vi "Generate Callchain.vi"() -> (3 "Callchain":string)   [LabVIEW 2020, in "hse-logger.lvlib" / "LogRecord.lvclass"]
doc: "Generates a easy to read callchain. Entries from the hse-logger.lvlib are ignored.\n\n____\nHAMPEL SOFTWARE ENGINEERING v2.0.6 (2021-04-15 11:38)"
uses:
  LogRecord.lvclass
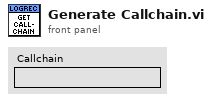
[diagram p1: front panel]
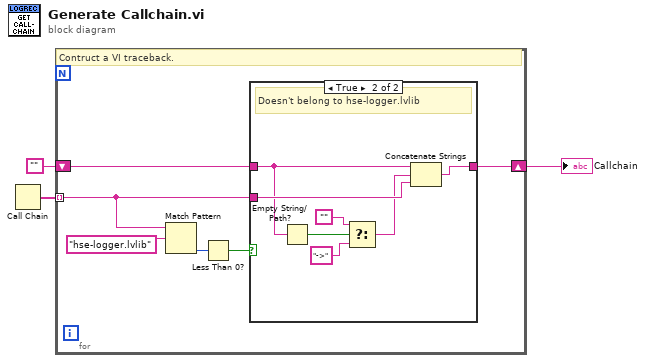
[diagram p0: block diagram]
diagram:
  n1 = Call Chain() -> (call chain=w2:string[])
  n2 = for {
    tunnel: w2 -> [w4] mode=indexing
    shift-right: [w8] -> w3
    shift-left: "" -> [w9]
    # "Contruct a VI traceback."
    n3 = Match Pattern(string=w4, regular expression="hse-logger.lvlib") -> (offset past match=w6:i32)  [unwired: 1 in, 3 out]
    n4 = Less Than 0?(x=w6) -> (x < 0?=w5:bool)
    n5 = case shown="True" w5 {
      tunnel: w9 -> [w10 w15]
      tunnel: [w10 w17] -> w8
      tunnel: w4 -> [_ w16]
      frame False {
        # "hse-logger.lvlib entry, don't add\nit to the callchain."
      }
      frame True {
        # "Doesn't belong to hse-logger.lvlib"
        n6 = Empty String/Path?(string/path=w15) -> (empty?=w14:bool)
        n7 = Select(t="", s=w14, f="->") -> (s? t:f=w13:string)
        n8 = Concatenate Strings(w15, w13, w16) -> (w17:string)
      }
    }
  }
  "Callchain" <- w3
